vi "Motor Multiplexer-DM.vi"(0 "Input of Motor Multiplexer":T1={"Mode"=1, "Direction"=FALSE, "Motor"=1, "Power"=100} {"Power" max=100 step=1; "Motor" min=1 max=4 step=1; "Mode" items=["RUN", "FLT", "BRK"]}, 2 "NXT":T2={"Hardware"="NXT", "Flattened String"=""}, 3 "Input Port":T3 items=["Port 1", "Port 2", "Port 3", "Port 4"]) -> (1 "Output of Motor Multiplexer":cluster{"Status":bool}, 4 "NXT dup":T2={"Hardware"="NXT", "Flattened String"=""} caption="NXT")   [LabVIEW 2011]
uses:
  <vilib>/NXT/Block Support/NXT_InputPort.ctl
  <vilib>/NXT/Subs/LVHSConnector.ctl
  <vilib>/NXT/Block Support/HWPage.SensorType.ctl
  <vilib>/NXT/Block Support/HWPage.SensorMode.ctl
panel:
  out "Status":bool caption="Success?"
  in  "Motormux address":u8=180 caption="Motormux Address" format="%x"
  # "mindsensors.com\nCopyright (c) 2009 by mindsensors.com\nEmail: info (<at>) mindsensors (<dot>) com\n\nThis program is free software. You can redistribute it and/or modify\nit under the terms of the GNU General Public License as published by\nthe Free Software Foundation; version 3 of the License.\nRead the license at: http://www.gnu.org/licenses/gpl.txt"
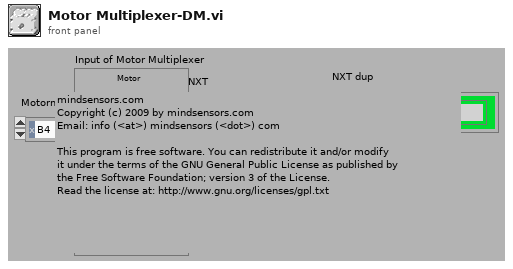
[diagram p1: front panel]
types:
  T1 = cluster{"Mode":u8, "Direction":bool, "Motor":u8, "Power":u8}
  T2 = typedef "LVHSConnector.ctl" = cluster{"Hardware":string, "Flattened String":string}
  T3 = typedef "NXT_InputPort.ctl" = u8
  T4 = typedef "HWPage.SensorType.ctl" = u8
  T5 = typedef "HWPage.SensorMode.ctl" = u8
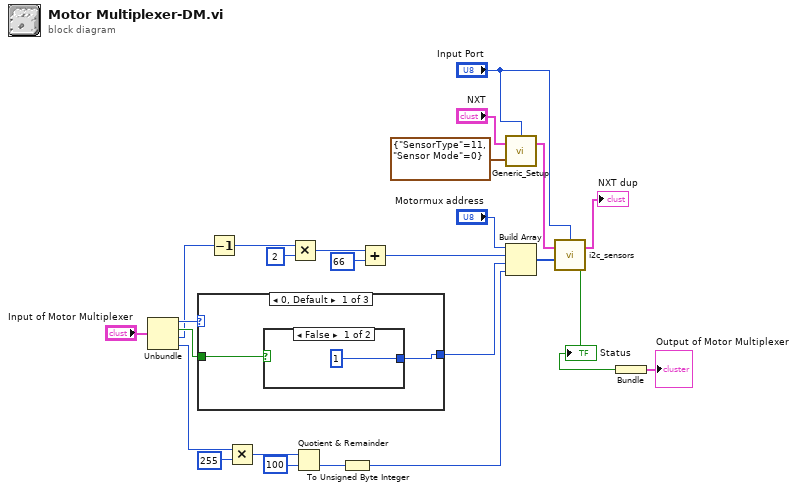
[diagram p0: block diagram]
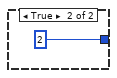
[diagram p2: hidden frame]
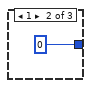
[diagram p3: hidden frame]
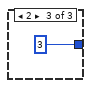
[diagram p4: hidden frame]
diagram:
  n1 = Unbundle("Input of Motor Multiplexer") -> ("Mode"=w6:u8, "Direction"=w5:bool, "Motor"=w4:u8, "Power"=w3:u8)
  n2 = case shown="0, Default" w6 {
    tunnel: [w27 0 3] -> w21
    tunnel: w5 -> [w26 _ _]
    frame 0, Default {
      n3 = case shown="False" w26 {
        tunnel: [1 2] -> w27
        frame False {
        }
        frame True {
        }
      }
    }
    frame 1 {
    }
    frame 2 {
    }
  }
  n4 = Decrement(x=w4) -> (x-1=w25:u8)
  n5 = Multiply(x=w3, y=u16 255) -> (x*y=w12:u16)
  n6 = Multiply(x=w25, y=u8 2) -> (x*y=w22:u8)
  n7 = Quotient & Remainder(x=w12, y=u16 100) -> (floor(x/y)=w10:u16)  [unwired: 1 out]
  n8 = To Unsigned Byte Integer(number=w10) -> (unsigned 8bit integer=w9:u8)
  n9 = Add(x=w22, y=u8 66 ("register")) -> (x+y=w15:u8)
  n10 = call <vilib>:"Generic_Setup.vi"("Sensor Setup"=cluster{"SensorType":T4, "Sensor Mode":T5} {"SensorType"=11, "Sensor Mode"=0}, "NXT"="NXT", "Port"="Input Port") -> ("NXT"=w18:T2)  [unwired: 1 out]
  n11 = Build Array("Motormux address", w15, w21, w9) -> (w14:i32[])
  n12 = call <vilib>:"i2c_sensors.vi"("Bytes to Write"=w14, "NXT"=w18, "Port"="Input Port") -> ("Success?"=w2:bool, "NXT"=→"NXT dup":T2)  [unwired: 2 in, 1 out]
  "Status" <- w2
  n13 = Bundle("Success?"=w2) -> (→"Output of Motor Multiplexer":cluster{"Success?":bool})  [unwired: 1 in]
